vi "GlobalStop.vi"() -> ()   [LabVIEW 2013]
panel:
  in  "STOP":bool
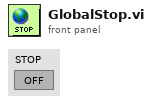
[diagram p1: front panel]
diagram:
